vi "Setup RT Configuration.vi"(7 "Virtual Memory Unit in":refnum<class "Virtual Memory Unit.lvclass">, 8 "error in (no error)":errorcluster, 11 "Remote Terminal in":refnum<class "Remote Terminal.lvclass">) -> (0 "error out":errorcluster, 3 "Remote Terminal out":refnum<class "Remote Terminal.lvclass">, 5 "Virtual Memory Unit out":refnum<class "Virtual Memory Unit.lvclass">)   [LabVIEW 2020, in "BCI-1553 API.lvlib" / "Remote Terminal.lvclass"]
doc: "Sets up all the configuration values for this Remote Terminal. All values are 'OR' masked into their proper locations in the resultant U16."
uses:
  Remote Terminal.lvclass
  Dependencies/Virtual Memory Unit/Virtual Memory Unit.lvclass
  Remote Terminal.lvclass/Remote Terminal.ctl
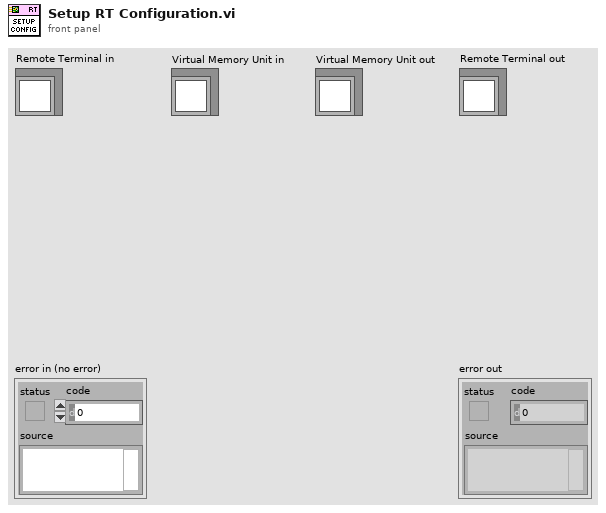
[diagram p1: front panel]
types:
  T1 = typedef "BCI-1553 API.lvlib/Remote Terminal.lvclass/Mode Code 17 Sync Configuration.ctl" = enum16{"Sync if Bit 0 = 1", "Sync if Bit 0 = 0", "Sync Unconditionally"}
  T2 = typedef "BCI-1553 API.lvlib/Remote Terminal.lvclass/RT-RT Timeout.ctl" = enum16{"57us", "62us", "100us", "180us"}
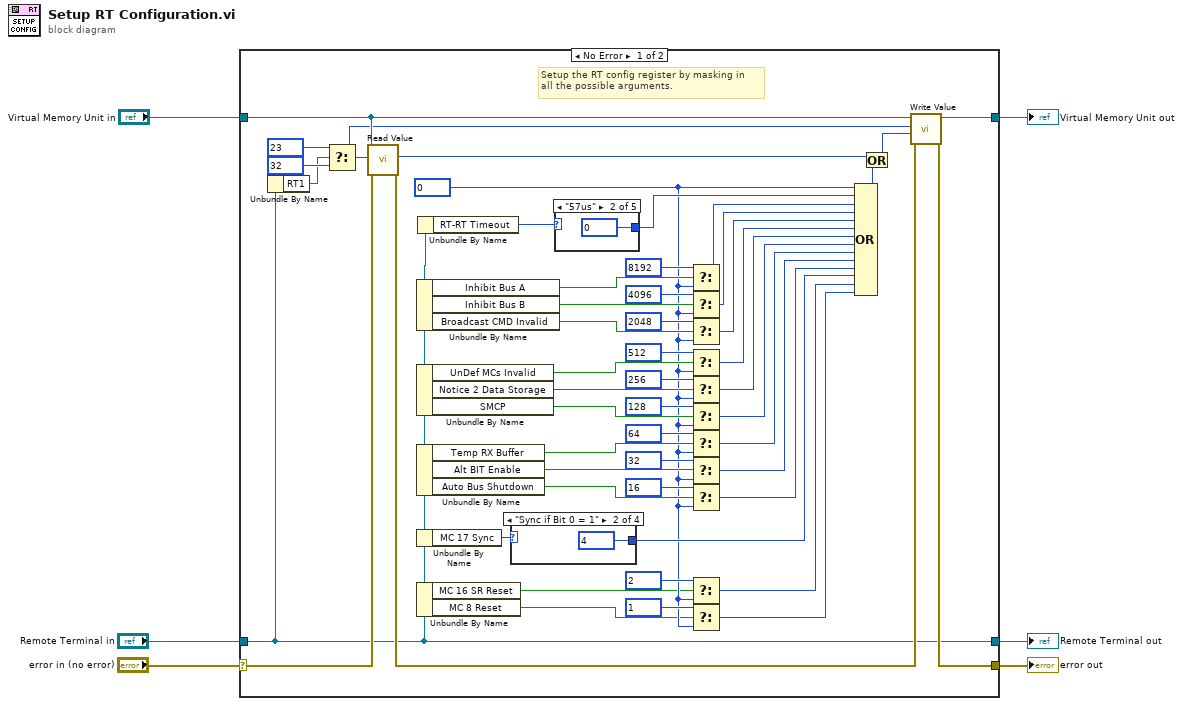
[diagram p0: block diagram]
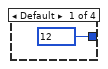
[diagram p2: hidden frame]
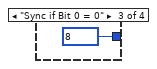
[diagram p3: hidden frame]
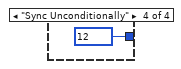
[diagram p4: hidden frame]
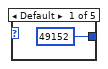
[diagram p5: hidden frame]
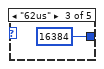
[diagram p6: hidden frame]
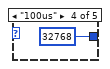
[diagram p7: hidden frame]
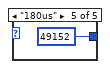
[diagram p8: hidden frame]
diagram:
  n1 = case shown="No Error" "error in (no error)" {
    selector: "error in (no error)" -> [w52 w69]
    tunnel: [w50 w69] -> w5
    tunnel: [w14 w68] -> w3
    tunnel: "Remote Terminal in" -> [w14 w68]
    tunnel: "Virtual Memory Unit in" -> [w53 w67]
    tunnel: [w8 w67] -> w1
    frame No Error {
      w15 = u16 0 ("Address")
      # "Setup the RT config register by masking in\nall the possible arguments."
      n2 = Unbundle By Name(w14) -> ("RT1"=w55:bool)
      n3 = Select(t=23 ("Address"), s=w55, f=32 ("Address")) -> (s? t:f=w7:i32)
      n4 = call "Read Value.vi"("error in (no error)"=w52, "Index"=w7, "Virtual Memory Unit in"=w53) -> ("error out"=w51:errorcluster, "Value"=w9:u16)  [unwired: 7 in]
      n5 = Unbundle By Name(w14) -> ("Inhibit Bus A"=w46:bool, "Inhibit Bus B"=w44:bool, "Broadcast CMD Invalid"=w40:bool)
      n6 = Unbundle By Name(w14) -> ("UnDef MCs Invalid"=w33:bool, "Notice 2 Data Storage"=w34:bool, "SMCP"=w32:bool)
      n7 = Unbundle By Name(w14) -> ("Temp RX Buffer"=w24:bool, "Alt BIT Enable"=w25:bool, "Auto Bus Shutdown"=w23:bool)
      n8 = Unbundle By Name(w14) -> ("MC 17 Sync"=w19:T1)
      n9 = Unbundle By Name(w14) -> ("MC 16 SR Reset"=w13:bool, "MC 8 Reset"=w12:bool)
      n10 = Unbundle By Name(w14) -> ("RT-RT Timeout"=w49:T2)
      n11 = case shown="\"Sync if Bit 0 = 1\"" w19 {
        tunnel: [u16 12 ("Address") u16 4 ("Address") u16 8 ("Address") u16 12 ("Address")] -> w18
        frame Default {
        }
        frame "Sync if Bit 0 = 1" {
        }
        frame "Sync if Bit 0 = 0" {
        }
        frame "Sync Unconditionally" {
        }
      }
      n12 = case shown="\"57us\"" w49 {
        tunnel: [u16 49152 ("Address") u16 0 ("Address") u16 16384 ("Address") u16 32768 ("Address") u16 49152 ("Address")] -> w47
        frame Default {
        }
        frame "57us" {
        }
        frame "62us" {
        }
        frame "100us" {
        }
        frame "180us" {
        }
      }
      n13 = Select(t=u16 8192 ("Address"), s=w46, f=w15) -> (s? t:f=w41:u16)
      n14 = Select(t=u16 4096 ("Address"), s=w44, f=w15) -> (s? t:f=w42:u16)
      n15 = Select(t=u16 2048 ("Address"), s=w40, f=w15) -> (s? t:f=w38:u16)
      n16 = Select(t=u16 512 ("Address"), s=w33, f=w15) -> (s? t:f=w31:u16)
      n17 = Select(t=u16 256 ("Address"), s=w34, f=w15) -> (s? t:f=w30:u16)
      n18 = Select(t=u16 128 ("Address"), s=w32, f=w15) -> (s? t:f=w29:u16)
      n19 = Select(t=u16 64 ("Address"), s=w24, f=w15) -> (s? t:f=w22:u16)
      n20 = Select(t=u16 32 ("Address"), s=w25, f=w15) -> (s? t:f=w21:u16)
      n21 = Select(t=u16 16 ("Address"), s=w23, f=w15) -> (s? t:f=w20:u16)
      n22 = Select(t=u16 2 ("Address"), s=w13, f=w15) -> (s? t:f=w11:u16)
      n23 = Select(t=u16 1 ("Address"), s=w12, f=w15) -> (s? t:f=w10:u16)
      n24 = Compound Arithmetic op=OR(w15, w47, w41, w42, w38, w31, w30, w29, w22, w21, w20, w18, w11, w10) -> (w48:u16)
      n25 = Or(x=w9, y=w48) -> (x .or. y?=w54:u16)
      n26 = call "Write Value.vi"("error in (no error)"=w51, "Value"=w54, "Index"=w7, "Virtual Memory Unit in"=w53) -> ("error out"=w50:errorcluster, "Virtual Memory Unit out"=w8:refnum<class "Virtual Memory Unit.lvclass">)  [unwired: 6 in]
    }
    frame Error {
    }
  }
  "error out" <- w5
  "Remote Terminal out" <- w3
  "Virtual Memory Unit out" <- w1
